vi "Set Pixel Resolution Unit.vi"(0 "Image Data in":u8[](array[numeric]), 1 "Im_File_Dir Offs":i32, 3 "Unit":u32(ring)=3 items=["None"=1, "Inch"=2, "Centimeter"=3], 4 "Litt/BigEnd":bool) -> (5 "Image Data out":u8[](array[numeric]))   [LabVIEW 2013, in "Tiff reader.lvlib"]
doc: "Sets the Pixel Resolution Tag in the Tiff file."
uses:
  Tiff reader.lvlib
  U16ToType.vi
  Long word to bytes.vi
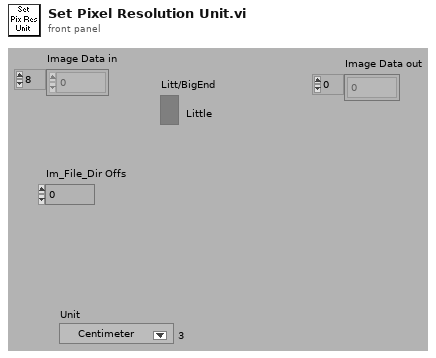
[diagram p1: front panel]
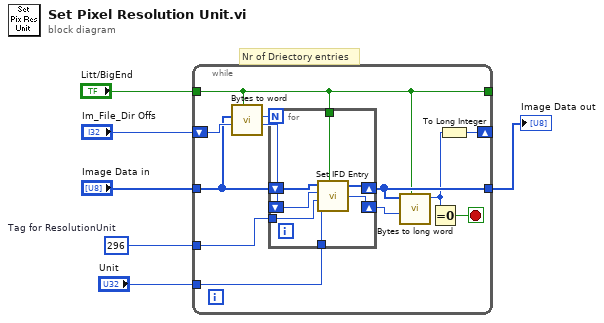
[diagram p0: block diagram]
diagram:
  w2 = u16 296  # Tag for ResolutionUnit
  # "Nr of Driectory entries"
  n1 = while {
    tunnel: "Image Data in" -> [w11]
    tunnel: [w16] -> w3
    shift-right: [w12] -> _
    shift-left: "Im_File_Dir Offs" -> [w18]
    tunnel: "Litt/BigEnd" -> [w9]
    tunnel: [w9] -> _
    tunnel: w2 -> [w8]
    tunnel: "Unit" -> [w7]
    stop <- w14 stop-if-true
    n2 = call "Bytes to word.vi"("Litt/BigEnd"=w9, "Index"=w18, "Image Data in"=w11) -> ("Index+2"=w17:i32, "Word"=w10:u16)  [unwired: 1 in, 4 out]
    n3 = for {
      N: w10 -> [_]
      shift-right: [w24] -> w16
      shift-left: w11 -> [w25]
      shift-right: [w21] -> w15
      shift-left: w17 -> [w23]
      tunnel: w9 -> [w22]
      tunnel: w8 -> [w20]
      tunnel: w7 -> [w19]
      n4 = call "Set IFD Entry.vi"("Image Data in"=w25, "Offset in"=w23, "Tag"=w20, "Val / Offset"=w19, "Litt/BigEnd"=w22) -> ("Image Data Out"=w24:u8[], "Directory Offset Out"=w21:i32)  [unwired: 1 out]
    }
    n5 = call "Bytes to long word.vi"("Litt/BigEnd"=w9, "Index"=w15, "Image Data in"=w16) -> ("U32"=w13:u32)  [unwired: 6 out]
    n6 = Equal To 0?(x=w13) -> (x = 0?=w14:bool)
    n7 = To Long Integer(number=w13) -> (32bit integer=w12:i32)
  }
  "Image Data out" <- w3
